vi "Get Data.vi"(8 "error in":errorcluster, 11 "eCRDS in":refnum<class "eCRDS.lvclass">) -> (0 "error out":errorcluster, 3 "eCRDS out":refnum<class "eCRDS.lvclass">)   [LabVIEW 2014, in "eCRDS Library.lvlib" / "eCRDS.lvclass"]
doc: "The base CRD <b>Get Data</b> implementation only handles the coadding of traces. If the property <b>Coadd</b> == 1, then this VI will do nothing."
uses:
  eCRDS.lvclass
  eCRDS.lvclass/eCRDS.ctl
  reusable/CRDS/Cell/CRDS Cell.lvclass/CRDS Cell.ctl
  reusable/General/Math/Fit Exponential Class/Fit Exponential.lvclass/Fit Exponential.ctl
  reusable/Instrument/Instrument.lvclass/Instrument.ctl
  reusable/CRDS/Cell/Write Laser Data.vi
  reusable/CRDS/Cell/Read Data.vi
  reusable/CRDS/Cell/Write Data.vi
  reusable/CRDS/Cell/Read ExpFit.vi
  reusable/General/Math/Fit Exponential Class/Set Dt.vi
  reusable/CRDS/Cell/Write ExpFit.vi
  <vilib>/DAQmx/read.llb/DAQmx Read (Analog 2D I16 NChan NSamp).vi
  reusable/CRDS/Main/Read Cells.vi
  reusable/Data/Write measTime.vi
  reusable/CRDS/Main/Write Cells.vi
  reusable/CRDS/Cell/CRDS Cell.lvclass
  reusable/CRDS/Data/Cell/CRDS Cell Data.lvclass
  reusable/General/Math/Fit Exponential Class/Fit Exponential.lvclass
  reusable/Instrument/Instrument.lvclass
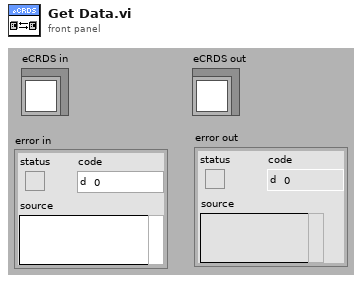
[diagram p1: front panel]
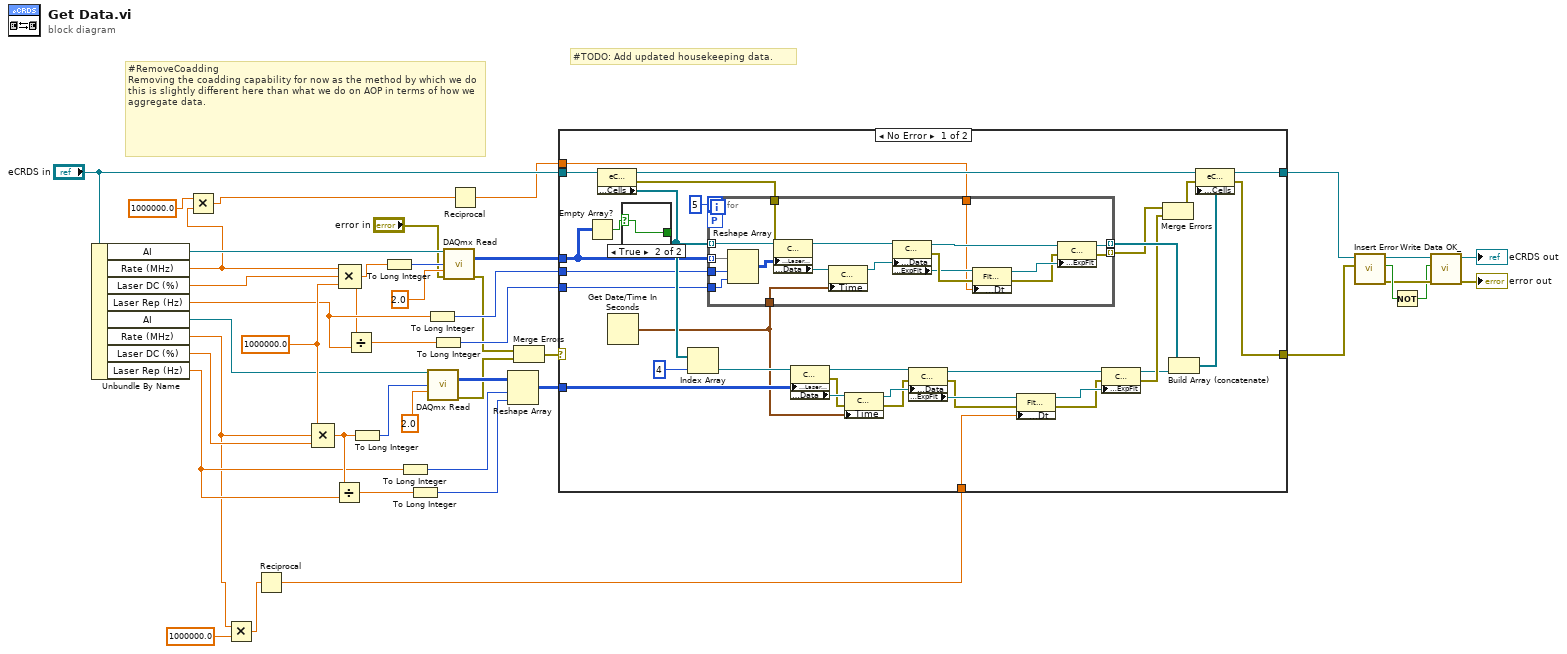
[diagram p0: block diagram]
diagram:
  w35 = 1000000.0 ("value")
  # "#TODO: Add updated housekeeping data."
  # "#RemoveCoadding\nRemoving the coadding capability for now as the method by which we do this is slightly different here than what we do on AOP in terms of how we aggregate data."
  n1 = Unbundle By Name("eCRDS in") -> ("AI"=w40:refnum<k21>, "Rate (MHz)"=w3:dbl, "Laser DC (%)"=w39:dbl, "Laser Rep (Hz)"=w31:dbl, "AI"=w34:refnum<k21>, "Rate (MHz)"=w6:dbl, "Laser DC (%)"=w22:dbl, "Laser Rep (Hz)"=w21:dbl)
  n2 = Multiply(x=1000000.0 ("y"), y=w3) -> (x*y=w1:dbl)
  n3 = Multiply(x=w6, y=1000000.0) -> (x*y=w4:dbl)
  n4 = Reciprocal(x=w4) -> (1/x=w8:dbl)
  n5 = Compound Arithmetic op=MULTIPLY(w35, w6, w22) -> (w26:dbl)
  n6 = Divide(x=w26, y=w21) -> (x/y=w28:dbl)
  n7 = Compound Arithmetic op=MULTIPLY(w3, w39, w35) -> (w24:dbl)
  n8 = Divide(x=w24, y=w31) -> (x/y=w33:dbl)
  n9 = To Long Integer(number=w26) -> (32bit integer=w25:i32)
  n10 = To Long Integer(number=w24) -> (32bit integer=w23:i32)
  n11 = To Long Integer(number=w21) -> (32bit integer=w29:i32)
  n12 = To Long Integer(number=w28) -> (32bit integer=w27:i32)
  n13 = To Long Integer(number=w31) -> (32bit integer=w30:i32)
  n14 = call-poly <vilib>:"DAQmx Read.vi"("task/channels in"=w34, "number of samples per channel"=w25, "timeout"=2.0) -> ("data"=w37:i16[][], "error out"=w19:errorcluster)  [unwired: 10 in, 1 out]
  n15 = To Long Integer(number=w33) -> (32bit integer=w32:i32)
  n16 = call-poly <vilib>:"DAQmx Read.vi"("task/channels in"=w40, "number of samples per channel"=w23, "timeout"=2.0, "error in"="error in") -> ("data"=w38:i16[][], "error out"=w20:errorcluster)  [unwired: 9 in, 1 out]
  n17 = Reciprocal(x=w1) -> (1/x=w7:dbl)
  n18 = Reshape Array(w37, w29, w27) -> (w36:i16[][])
  n19 = Merge Errors(w20, w19) -> (w18:errorcluster)
  n20 = case shown="No Error" w18 {
    selector: w18 -> [_ w97]
    tunnel: [w76 w98] -> w15
    tunnel: w38 -> [w45 _]
    tunnel: "eCRDS in" -> [w75 w98]
    tunnel: w36 -> [w70 _]
    tunnel: w32 -> [w66 _]
    tunnel: w30 -> [w65 _]
    tunnel: [w61 w97] -> w16
    tunnel: w8 -> [w52 _]
    tunnel: w7 -> [w46 _]
    frame No Error {
      n21 = Empty Array?(array=w45) -> (empty?=w44:bool)
      n22 = property class="eCRDS"(reference=w75) -> (reference out=w74:refnum<class "eCRDS.lvclass">, error out=w64:errorcluster, "Data Access:Cells"=w72:refnum<class "CRDS Cell.lvclass">[])  [unwired: 1 in]
      n23 = Get Date/Time In Seconds() -> (seconds since 1Jan1904=w57:timestamp)
      n24 = case shown="True" w44 {
        selector: w44 -> [w77 w78]
        tunnel: [w77 w78] -> _
        frame False {
        }
        frame True {
        }
      }
      n25 = Index Array(array=w72, index=4) -> (element=w69:refnum<class "CRDS Cell.lvclass">)
      n26 = for {
        N: 5 -> [_]
        tunnel: w45 -> [w96] mode=indexing
        tunnel: w66 -> [w94]
        tunnel: w65 -> [w95]
        tunnel: w72 -> [w93] mode=indexing
        tunnel: [w80] -> w68 mode=indexing
        workers-P: _ -> [_]
        tunnel: w64 -> [w91]
        tunnel: [w79] -> w63 mode=indexing
        tunnel: w57 -> [w87]
        tunnel: w46 -> [w81]
        n27 = Reshape Array(w96, w95, w94) -> (w92:i16[][])
        n28 = property class="CRDS Cell"(reference=w93, error in=w91, "Accessors:Laser Data"=w92) -> (reference out=w90:refnum<class "CRDS Cell.lvclass">, "Data Access:Data"=w89:refnum<class "CRDS Cell Data.lvclass">)  [unwired: 1 out]
        n29 = property class="CRDS Cell"(reference=w89, "Time"=w87) -> (reference out=w88:refnum<class "CRDS Cell Data.lvclass">)  [unwired: 1 in, 1 out]
        n30 = property class="CRDS Cell"(reference=w90, "Data Access:Data"=w88) -> (reference out=w84:refnum<class "CRDS Cell.lvclass">, error out=w83:errorcluster, "Data Access:ExpFit"=w82:refnum<class "Fit Exponential.lvclass">)  [unwired: 1 in]
        n31 = property class="Fit Exp"(reference=w82, error in=w83, "Accessors:Dt"=w81) -> (reference out=w86:refnum<class "Fit Exponential.lvclass">, error out=w85:errorcluster)
        n32 = property class="CRDS Cell"(reference=w84, error in=w85, "Data Access:ExpFit"=w86) -> (reference out=w80:refnum<class "CRDS Cell.lvclass">, error out=w79:errorcluster)
      }
      n33 = property class="CRDS Cell"(reference=w69, "Accessors:Laser Data"=w70) -> (reference out=w59:refnum<class "CRDS Cell.lvclass">, error out=w56:errorcluster, "Data Access:Data"=w58:refnum<class "CRDS Cell Data.lvclass">)  [unwired: 1 in]
      n34 = property class="CRDS Cell"(reference=w58, error in=w56, "Time"=w57) -> (reference out=w60:refnum<class "CRDS Cell Data.lvclass">, error out=w55:errorcluster)
      n35 = property class="CRDS Cell"(reference=w59, error in=w55, "Data Access:Data"=w60) -> (reference out=w51:refnum<class "CRDS Cell.lvclass">, error out=w53:errorcluster, "Data Access:ExpFit"=w54:refnum<class "Fit Exponential.lvclass">)
      n36 = property class="Fit Exp"(reference=w54, error in=w53, "Accessors:Dt"=w52) -> (reference out=w50:refnum<class "Fit Exponential.lvclass">, error out=w49:errorcluster)
      n37 = property class="CRDS Cell"(reference=w51, error in=w49, "Data Access:ExpFit"=w50) -> (reference out=w47:refnum<class "CRDS Cell.lvclass">, error out=w48:errorcluster)
      n38 = Merge Errors(w63, w48) -> (w62:errorcluster)
      n39 = Build Array (concatenate)(w68, w47) -> (w67:refnum<class "CRDS Cell.lvclass">[])
      n40 = property class="eCRDS"(reference=w74, error in=w62, "Data Access:Cells"=w67) -> (reference out=w76:refnum<class "eCRDS.lvclass">, error out=w61:errorcluster)
    }
    frame Error {
    }
  }
  n41 = call "Insert Error.vi"("err"=w16, "Instrument in"=w15) -> ("error out"=w12:errorcluster, "error?"=w13:bool, "Instrument out"=w14:refnum<class "eCRDS.lvclass">)  [unwired: 7 in]
  n42 = Not(x=w13) -> (.not. x?=w9:bool)
  n43 = call "Write Data OK_.vi"("error in (no error)"=w12, "Data OK?"=w9, "Instrument in"=w14) -> ("error out"=→"error out":errorcluster, "Instrument out"=→"eCRDS out":refnum<class "eCRDS.lvclass">)  [unwired: 7 in]
